vi "WaitForTransition.vi"(4 "error in (no error)":errorcluster, 7 "State":T1=enum."Initialising") -> (0 "error out":errorcluster, 3 "StateOut":T1=enum."Initialising")   [LabVIEW 2023]
doc: "*-----------------------------------------------------\n* Author: SWatts\n*\n* VI Description: Dependent on State will transition to a new state, uses StateQ\n* \n*\n* Error handling: All errors passed out\n*\n* Pre-condition: \n*\n* Post-condition: None\n*\n* Revision History:\n*\n* Rev Date Author Description \n* 01 30/04/2014 SWatts First issue\n*\n*-----------------------------------------------------"
uses:
  Controls/SetupModeState.ctl
  Controls/QueueCommand.ctl
panel:
  # "Output"
  # "Input"
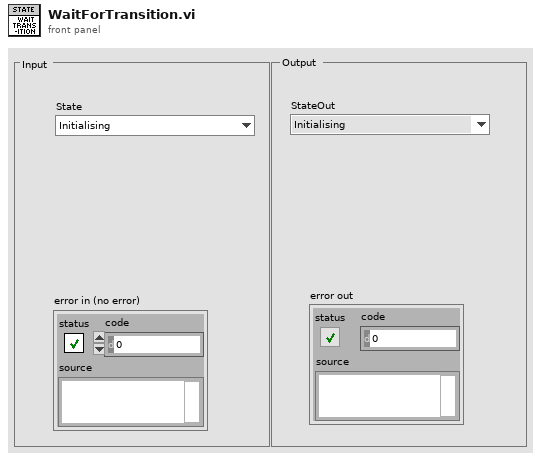
[diagram p1: front panel]
types:
  T1 = typedef "SetupModeState.ctl" = enum16{"No State - Error", "Initialising", "Idling", "Running", "Sorting Menu", "Resetting Menu", "Loading UI", "Erroring", "Exiting"}
  T2 = typedef "QueueCommand.ctl" = enum16{"No Command - Error", "Initialise", "Add to Bottom", "Add To Top", "Get Ref", "Close"}
  T3 = typedef "StateMessage.ctl" = cluster{"Transition":T4, "variant":variant}
  T4 = typedef "Transition.ctl" = enum16{"No Transition - Error", "Initialise", "Login", "Authenticate", "Log on Fail", "Login Success", "Logout", "Generate Error", "Start", "Stop", "Menu Button Pressed", "UI Button Pressed", "Exit"}
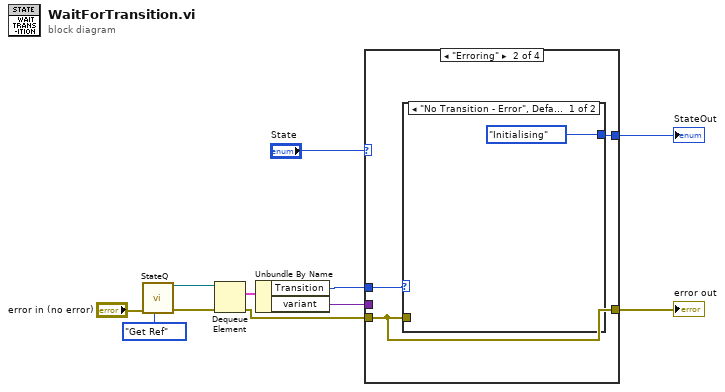
[diagram p0: block diagram]
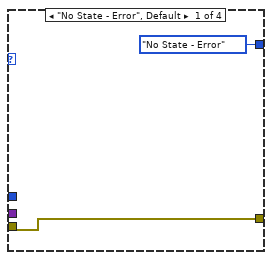
[diagram p2: hidden frame]
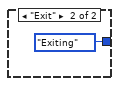
[diagram p3: hidden frame]
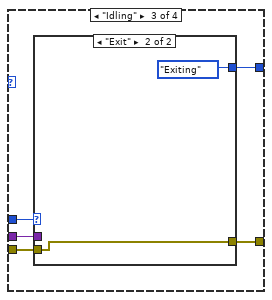
[diagram p4: hidden frame]
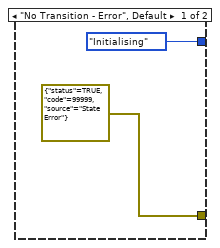
[diagram p5: hidden frame]
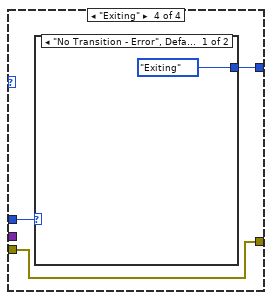
[diagram p6: hidden frame]
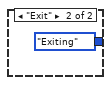
[diagram p7: hidden frame]
diagram:
  n1 = call "StateQ.vi"("QueueCommand"=QueueCommand."Get Ref", "error in (no error)"="error in (no error)") -> ("error out"=w6:errorcluster, "queue out"=w5:refnum<queue>)  [unwired: 5 in]
  n2 = Dequeue Element(queue=w5, error in (no error)=w6) -> (element=w11:T3, error out=w8:errorcluster)  [unwired: 1 in, 2 out]
  n3 = Unbundle By Name(w11) -> ("Transition"=w10:T4, "variant"=w9:variant)
  n4 = case shown="\"Erroring\"" "State" {
    tunnel: w10 -> [_ w16 w23 w30]
    tunnel: w9 -> [_ _ w22 _]
    tunnel: w8 -> [w12 w14 w21 w28]
    tunnel: [w12 w14 w20 w28] -> w3
    tunnel: [SetupModeState."No State - Error" ("State 2") w15 w19 w29] -> w2
    frame "No State - Error", Default {
    }
    frame "Erroring" {
      n5 = case shown="\"No Transition - Error\", Default" w16 {
        tunnel: [SetupModeState."Initialising" ("State 2") SetupModeState."Exiting" ("State 2")] -> w15
        tunnel: w14 -> [_ _]
        frame "No Transition - Error", Default {
        }
        frame "Exit" {
        }
      }
    }
    frame "Idling" {
      n6 = case shown="\"Exit\"" w23 {
        tunnel: w22 -> [_ _]
        tunnel: [SetupModeState."Initialising" ("State 2") SetupModeState."Exiting" ("State 2")] -> w19
        tunnel: w21 -> [_ w26]
        tunnel: [errorcluster {"status"=TRUE, "code"=99999, "source"="State Error"} ("error out") w26] -> w20
        frame "No Transition - Error", Default {
        }
        frame "Exit" {
        }
      }
    }
    frame "Exiting" {
      n7 = case shown="\"No Transition - Error\", Default" w30 {
        tunnel: [SetupModeState."Exiting" ("State 2") SetupModeState."Exiting" ("State 2")] -> w29
        frame "No Transition - Error", Default {
        }
        frame "Exit" {
        }
      }
    }
  }
  "error out" <- w3
  "StateOut" <- w2
